vi "notifyObservers.vi"(8 "error in (no error)":errorcluster, 11 "Observable in":refnum<class "Observable.lvclass">) -> (0 "error out":errorcluster, 3 "Observable out":refnum<class "Observable.lvclass">)   [LabVIEW 2020, in "Observable.lvclass"]
uses:
  Observable.lvclass
  Observer/Observer.lvclass
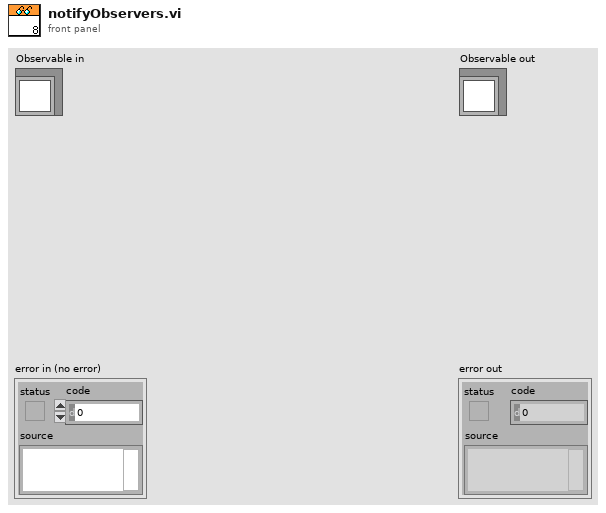
[diagram p1: front panel]
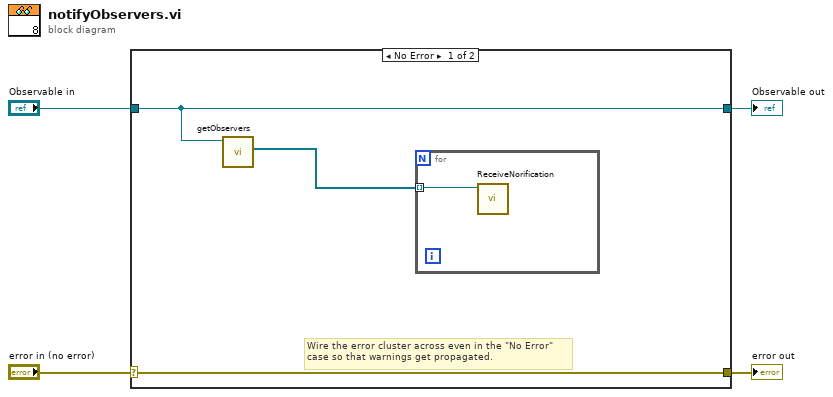
[diagram p0: block diagram]
diagram:
  n1 = case shown="No Error" "error in (no error)" {
    selector: "error in (no error)" -> [w7 w10]
    tunnel: [w7 w10] -> w3
    tunnel: [w5 w9] -> w1
    tunnel: "Observable in" -> [w5 w9]
    frame No Error {
      # "Wire the error cluster across even in the \"No Error\"\ncase so that warnings get propagated."
      n2 = call-dynamic "getObservers.vi"("Observable in"=w5) -> ("Observers"=w6:refnum<class "Observer.lvclass">[])  [unwired: 8 in, 2 out]
      n3 = for {
        tunnel: w6 -> [w8] mode=indexing
        n4 = call-dynamic "ReceiveNorification.vi"("Observer in"=w8) -> ()  [unwired: 9 in, 2 out]
      }
    }
    frame Error {
    }
  }
  "error out" <- w3
  "Observable out" <- w1
